vi "ConvertDiagPacket.vi"(8 "error in (no error)":errorcluster, 10 ".NET data in":refnum<k24>, 11 "controller in":refnum<k24>) -> (0 "error out":errorcluster, 2 "LabVIEW data out":T1, 3 "controller out":refnum<k24>)   [LabVIEW 2017]
uses:
  AxisDiagPacket.ctl
  ControllerDiagPacket.ctl
  C:/Users/OmerLab/Documents/GitHub/RamanSpecUsingStageXY/Bin/Aerotech.Ensemble.LabVIEW.dll
  Bin/Aerotech.Ensemble.LabVIEW.dll
  C:/Users/OmerLab/Documents/GitHub/RamanSpecUsingStageXY/Bin/Aerotech.Ensemble.dll
  Bin/Aerotech.Ensemble.dll
panel:
  in  "ControllerDiagPacket Type":T1
  in  "AxisDiagPacket Type":T2
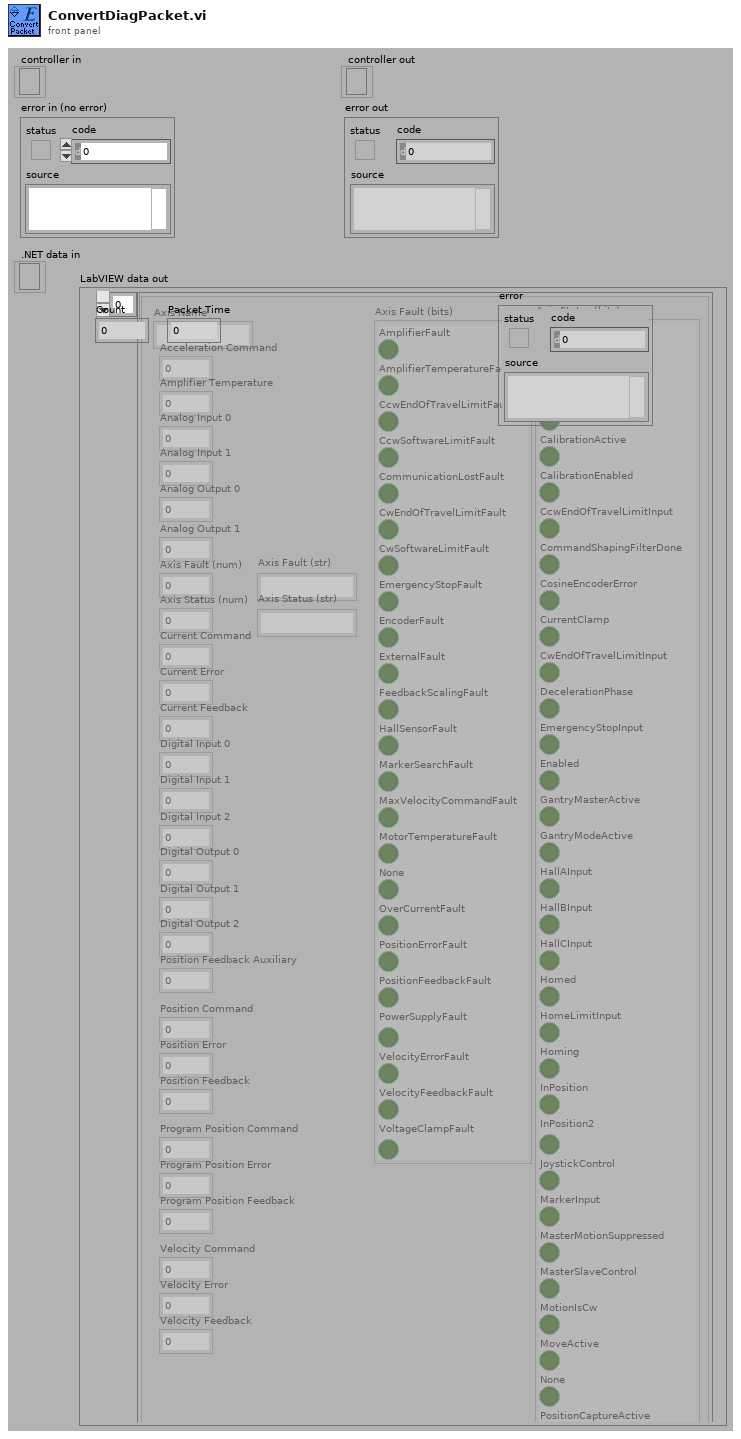
[diagram p1: front panel]
types:
  T1 = typedef "ControllerDiagPacket.ctl" = cluster{"Count":i32, "Packet Time":i64, "Axes":T2[], "error":errorcluster}
  T2 = typedef "AxisDiagPacket.ctl" = cluster{"Axis Name":string, "Acceleration Command":dbl, "Amplifier Temperature":sgl, "Analog Input 0":dbl, "Analog Input 1":dbl, "Analog Output 0":dbl, "Analog Output 1":dbl, "Axis Fault (num)":i32, "Axis Fault (str)":string, "Axis Fault (bits)":cluster{"AmplifierFault":bool, "AmplifierTemperatureFault":bool, "CcwEndOfTravelLimitFault":bool, "CcwSoftwareLimitFault":bool, "CommunicationLostFault":bool, "CwEndOfTravelLimitFault":bool, "CwSoftwareLimitFault":bool, "EmergencyStopFault":bool, "EncoderFault":bool, "ExternalFault":bool, "FeedbackScalingFault":bool, "HallSensorFault":bool, "MarkerSearchFault":bool, "MaxVelocityCommandFault":bool, "MotorTemperatureFault":bool, "None":bool, "OverCurrentFault":bool, "PositionErrorFault":bool, "PositionFeedbackFault":bool, "PowerSupplyFault":bool, "VelocityErrorFault":bool, "VelocityFeedbackFault":bool, "VoltageClampFault":bool}, "Axis Status (num)":i32, "Axis Status (str)":string, "Axis Status (bits)":cluster{"AccelerationPhase":bool, "AutofocusActive":bool, "BrakeOutput":bool, "CalibrationActive":bool, "CalibrationEnabled":bool, "CcwEndOfTravelLimitInput":bool, "CommandShapingFilterDone":bool, "CosineEncoderError":bool, "CurrentClamp":bool, "CwEndOfTravelLimitInput":bool, "DecelerationPhase":bool, "EmergencyStopInput":bool, "Enabled":bool, "GantryMasterActive":bool, "GantryModeActive":bool, "HallAInput":bool, "HallBInput":bool, "HallCInput":bool, "Homed":bool, "HomeLimitInput":bool, "Homing":bool, "InPosition":bool, "InPosition2":bool, "JoystickControl":bool, "MarkerInput":bool, "MasterMotionSuppressed":bool, "MasterSlaveControl":bool, "MotionIsCw":bool, "MoveActive":bool, "None":bool, "PositionCaptureActive":bool, "ServoControl":bool, "SineEncoderError":bool}, "Current Command":sgl, "Current Error":sgl, "Current Feedback":sgl, "Digital Input 0":i32, "Digital Input 1":i32, "Digital Input 2":i32, "Digital Output 0":i32, "Digital Output 1":i32, "Digital Output 2":i32, "Position Feedback Auxiliary":dbl, "Position Command":dbl, "Position Error":dbl, "Position Feedback":dbl, "Program Position Command":dbl, "Program Position Error":dbl, "Program Position Feedback":dbl, "Velocity Command":dbl, "Velocity Error":dbl, "Velocity Feedback":dbl}
  T3 = cluster{"AccelerationPhase":bool, "AutofocusActive":bool, "BrakeOutput":bool, "CalibrationActive":bool, "CalibrationEnabled":bool, "CcwEndOfTravelLimitInput":bool, "CommandShapingFilterDone":bool, "CosineEncoderError":bool, "CurrentClamp":bool, "CwEndOfTravelLimitInput":bool, "DecelerationPhase":bool, "EmergencyStopInput":bool, "Enabled":bool, "GantryMasterActive":bool, "GantryModeActive":bool, "HallAInput":bool, "HallBInput":bool, "HallCInput":bool, "Homed":bool, "HomeLimitInput":bool, "Homing":bool, "InPosition":bool, "InPosition2":bool, "JoystickControl":bool, "MarkerInput":bool, "MasterMotionSuppressed":bool, "MasterSlaveControl":bool, "MotionIsCw":bool, "MoveActive":bool, "None":bool, "PositionCaptureActive":bool, "ServoControl":bool, "SineEncoderError":bool}
  T4 = cluster{"AmplifierFault":bool, "AmplifierTemperatureFault":bool, "CcwEndOfTravelLimitFault":bool, "CcwSoftwareLimitFault":bool, "CommunicationLostFault":bool, "CwEndOfTravelLimitFault":bool, "CwSoftwareLimitFault":bool, "EmergencyStopFault":bool, "EncoderFault":bool, "ExternalFault":bool, "FeedbackScalingFault":bool, "HallSensorFault":bool, "MarkerSearchFault":bool, "MaxVelocityCommandFault":bool, "MotorTemperatureFault":bool, "None":bool, "OverCurrentFault":bool, "PositionErrorFault":bool, "PositionFeedbackFault":bool, "VelocityErrorFault":bool, "VelocityFeedbackFault":bool, "VoltageClampFault":bool, "PowerSupplyFault":bool}
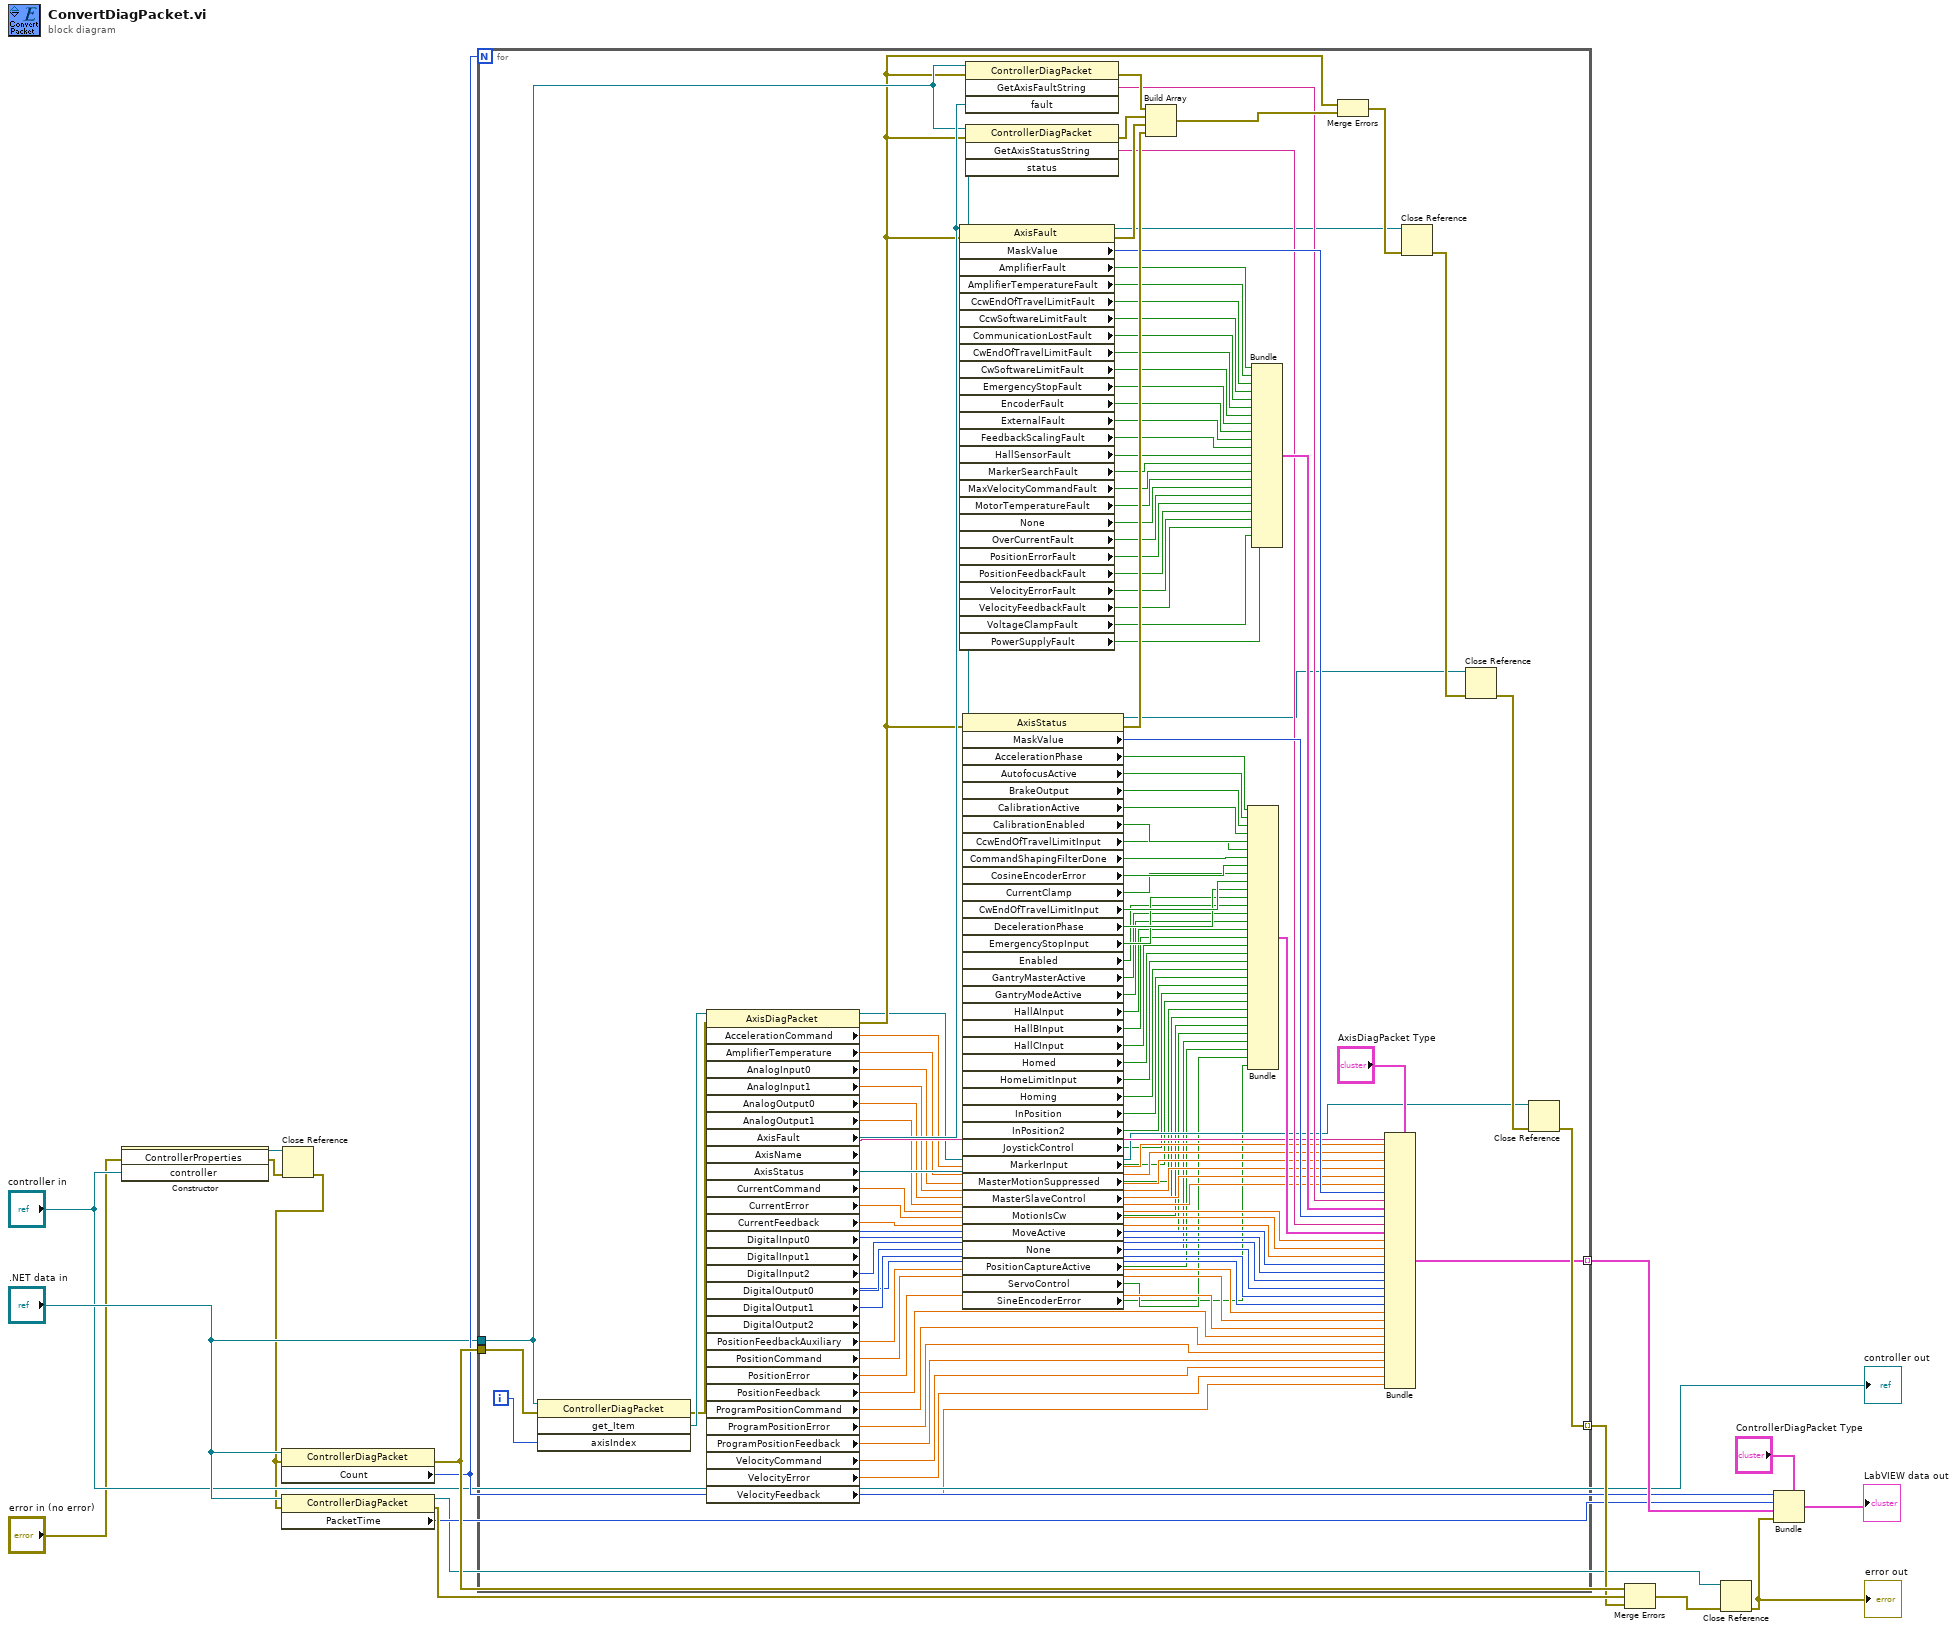
[diagram p0: block diagram]
diagram:
  n1 = constructor class="ControllerProperties"(error in="error in (no error)", "controller"="controller in") -> (reference out=w3:refnum<k24>, error out=w1:errorcluster)  [unwired: 2 in, 2 out]
  n2 = Close Reference(reference=w3, error in (no error)=w1) -> (error out=w2:errorcluster)
  n3 = property class="ControllerDiagPacket"(reference=".NET data in", error in=w2) -> (error out=w16:errorcluster, "Count"=w12:i32)  [unwired: 1 out]
  n4 = property class="ControllerDiagPacket"(reference=".NET data in", error in=w2) -> (reference out=w6:refnum<k24>, error out=w17:errorcluster, "PacketTime"=w13:i64)
  n5 = for {
    N: w12 -> [_]
    tunnel: [w91] -> w14 mode=indexing
    tunnel: w16 -> [w126]
    tunnel: ".NET data in" -> [w115]
    tunnel: [w97] -> w15 mode=indexing
    i -> [w127]
    n6 = invoke class="ControllerDiagPacket" method="get_Item"(reference=w115, error in=w126, "axisIndex"=w127) -> (error out=w124:errorcluster, "get_Item"=w125:refnum<k24>)  [unwired: 1 in, 2 out]
    n7 = property class="AxisDiagPacket"(reference=w125, error in=w124) -> (reference out=w62:refnum<k24>, error out=w69:errorcluster, "AccelerationCommand"=w68:dbl, "AmplifierTemperature"=w67:sgl, "AnalogInput0"=w66:dbl, "AnalogInput1"=w65:dbl, "AnalogOutput0"=w64:dbl, "AnalogOutput1"=w63:dbl, "AxisFault"=w117:refnum<k24>, "AxisName"=w79:string, "AxisStatus"=w116:refnum<k24>, "CurrentCommand"=w89:sgl, "CurrentError"=w88:sgl, "CurrentFeedback"=w87:sgl, "DigitalInput0"=w86:i32, "DigitalInput1"=w85:i32, "DigitalInput2"=w84:i32, "DigitalOutput0"=w83:i32, "DigitalOutput1"=w82:i32, "DigitalOutput2"=w81:i32, "PositionFeedbackAuxiliary"=w80:dbl, "PositionCommand"=w78:dbl, "PositionError"=w77:dbl, "PositionFeedback"=w76:dbl, "ProgramPositionCommand"=w75:dbl, "ProgramPositionError"=w74:dbl, "ProgramPositionFeedback"=w73:dbl, "VelocityCommand"=w72:dbl, "VelocityError"=w71:dbl, "VelocityFeedback"=w70:dbl)
    n8 = property class="AxisFault"(reference=w117, error in=w69) -> (reference out=w93:refnum<k24>, error out=w120:errorcluster, "MaskValue"=w118:i32, "AmplifierFault"=w42:bool, "AmplifierTemperatureFault"=w41:bool, "CcwEndOfTravelLimitFault"=w40:bool, "CcwSoftwareLimitFault"=w39:bool, "CommunicationLostFault"=w38:bool, "CwEndOfTravelLimitFault"=w37:bool, "CwSoftwareLimitFault"=w36:bool, "EmergencyStopFault"=w35:bool, "EncoderFault"=w34:bool, "ExternalFault"=w33:bool, "FeedbackScalingFault"=w32:bool, "HallSensorFault"=w31:bool, "MarkerSearchFault"=w30:bool, "MaxVelocityCommandFault"=w29:bool, "MotorTemperatureFault"=w28:bool, "None"=w27:bool, "OverCurrentFault"=w26:bool, "PositionErrorFault"=w25:bool, "PositionFeedbackFault"=w24:bool, "VelocityErrorFault"=w23:bool, "VelocityFeedbackFault"=w22:bool, "VoltageClampFault"=w19:bool, "PowerSupplyFault"=w18:bool)
    n9 = property class="AxisStatus"(reference=w116, error in=w69) -> (reference out=w92:refnum<k24>, error out=w119:errorcluster, "MaskValue"=w100:i32, "AccelerationPhase"=w114:bool, "AutofocusActive"=w113:bool, "BrakeOutput"=w112:bool, "CalibrationActive"=w111:bool, "CalibrationEnabled"=w110:bool, "CcwEndOfTravelLimitInput"=w109:bool, "CommandShapingFilterDone"=w108:bool, "CosineEncoderError"=w107:bool, "CurrentClamp"=w106:bool, "CwEndOfTravelLimitInput"=w105:bool, "DecelerationPhase"=w104:bool, "EmergencyStopInput"=w103:bool, "Enabled"=w61:bool, "GantryMasterActive"=w60:bool, "GantryModeActive"=w59:bool, "HallAInput"=w58:bool, "HallBInput"=w57:bool, "HallCInput"=w56:bool, "Homed"=w55:bool, "HomeLimitInput"=w54:bool, "Homing"=w53:bool, "InPosition"=w52:bool, "InPosition2"=w51:bool, "JoystickControl"=w50:bool, "MarkerInput"=w49:bool, "MasterMotionSuppressed"=w48:bool, "MasterSlaveControl"=w47:bool, "MotionIsCw"=w46:bool, "MoveActive"=w45:bool, "None"=w44:bool, "PositionCaptureActive"=w43:bool, "ServoControl"=w21:bool, "SineEncoderError"=w20:bool)
    n10 = invoke class="ControllerDiagPacket" method="GetAxisFaultString"(reference=w115, error in=w69, "fault"=w117) -> (error out=w123:errorcluster, "GetAxisFaultString"=w102:string)  [unwired: 1 in, 2 out]
    n11 = invoke class="ControllerDiagPacket" method="GetAxisStatusString"(reference=w115, error in=w69, "status"=w116) -> (error out=w121:errorcluster, "GetAxisStatusString"=w99:string)  [unwired: 1 in, 2 out]
    n12 = Build Array(w123, w121, w120, w119) -> (w122:errorcluster[])
    n13 = Bundle("AccelerationPhase"=w114, "AutofocusActive"=w113, "BrakeOutput"=w112, "CalibrationActive"=w111, "CalibrationEnabled"=w110, "CcwEndOfTravelLimitInput"=w109, "CommandShapingFilterDone"=w108, "CosineEncoderError"=w107, "CurrentClamp"=w106, "CwEndOfTravelLimitInput"=w105, "DecelerationPhase"=w104, "EmergencyStopInput"=w103, "Enabled"=w61, "GantryMasterActive"=w60, "GantryModeActive"=w59, "HallAInput"=w58, "HallBInput"=w57, "HallCInput"=w56, "Homed"=w55, "HomeLimitInput"=w54, "Homing"=w53, "InPosition"=w52, "InPosition2"=w51, "JoystickControl"=w50, "MarkerInput"=w49, "MasterMotionSuppressed"=w48, "MasterSlaveControl"=w47, "MotionIsCw"=w46, "MoveActive"=w45, "None"=w44, "PositionCaptureActive"=w43, "ServoControl"=w21, "SineEncoderError"=w20) -> (w98:T3)  [unwired: 1 in]
    n14 = Bundle("AmplifierFault"=w42, "AmplifierTemperatureFault"=w41, "CcwEndOfTravelLimitFault"=w40, "CcwSoftwareLimitFault"=w39, "CommunicationLostFault"=w38, "CwEndOfTravelLimitFault"=w37, "CwSoftwareLimitFault"=w36, "EmergencyStopFault"=w35, "EncoderFault"=w34, "ExternalFault"=w33, "FeedbackScalingFault"=w32, "HallSensorFault"=w31, "MarkerSearchFault"=w30, "MaxVelocityCommandFault"=w29, "MotorTemperatureFault"=w28, "None"=w27, "OverCurrentFault"=w26, "PositionErrorFault"=w25, "PositionFeedbackFault"=w24, "VelocityErrorFault"=w23, "VelocityFeedbackFault"=w22, "VoltageClampFault"=w19, "PowerSupplyFault"=w18) -> (w101:T4)  [unwired: 1 in]
    n15 = Merge Errors(w69, w122) -> (w94:errorcluster)
    n16 = Bundle(cluster="AxisDiagPacket Type", "Axis Name"=w79, "Acceleration Command"=w68, "Amplifier Temperature"=w67, "Analog Input 0"=w66, "Analog Input 1"=w65, "Analog Output 0"=w64, "Analog Output 1"=w63, "Axis Fault (num)"=w118, "Axis Fault (str)"=w102, "Axis Fault (bits)"=w101, "Axis Status (num)"=w100, "Axis Status (str)"=w99, "Axis Status (bits)"=w98, "Current Command"=w89, "Current Error"=w88, "Current Feedback"=w87, "Digital Input 0"=w86, "Digital Input 1"=w85, "Digital Input 2"=w84, "Digital Output 0"=w83, "Digital Output 1"=w82, "Digital Output 2"=w81, "Position Feedback Auxiliary"=w80, "Position Command"=w78, "Position Error"=w77, "Position Feedback"=w76, "Program Position Command"=w75, "Program Position Error"=w74, "Program Position Feedback"=w73, "Velocity Command"=w72, "Velocity Error"=w71, "Velocity Feedback"=w70) -> (w91:T2)
    n17 = Close Reference(reference=w93, error in (no error)=w94) -> (error out=w95:errorcluster)
    n18 = Close Reference(reference=w92, error in (no error)=w95) -> (error out=w96:errorcluster)
    n19 = Close Reference(reference=w62, error in (no error)=w96) -> (error out=w97:errorcluster)
  }
  n20 = Merge Errors(w16, w17, w15) -> (w8:errorcluster)
  n21 = Close Reference(reference=w6, error in (no error)=w8) -> (error out=w7:errorcluster)
  "error out" <- w7
  n22 = Bundle(cluster="ControllerDiagPacket Type", "Count"=w12, "Packet Time"=w13, "Axes"=w14, "error"=w7) -> (→"LabVIEW data out":T1)
  "controller out" <- "controller in"
